vi "SpeedAccelM1.vi"() -> ()   [LabVIEW 2015]
uses:
  <instrlib>/Ion Motion Roboclaw/Ion Motion Roboclaw.lvlib
panel:
  in  "Address":u8
  in  "stop":bool
  in  "Accel":u32(slide) max=800000 step=10000 scale=0.0..800000.0
  in  "Speed":i32(slide)=-40000 min=-40000 max=40000 step=1000 scale=-40000.0..40000.0
  out "Valid":bool
  out "error out":errorcluster
  in  "COM port":refnum<visa-resource-name>
  in  "baud rate (38400)":u32
  in  "error in (no error)":errorcluster
  # "This example assumes the Velocity PID  values have already been tuned for the motor and saved to the Roboclaw."
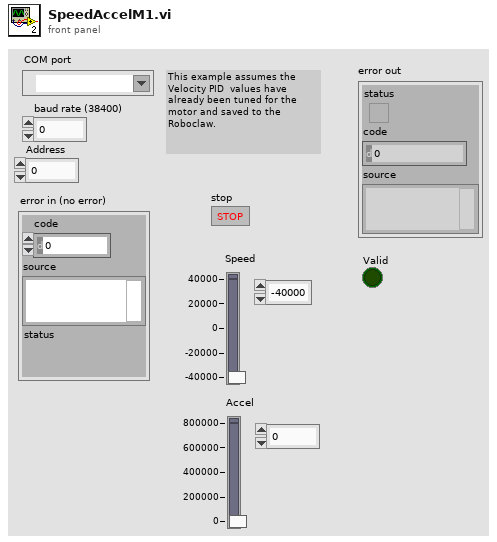
[diagram p1: front panel]
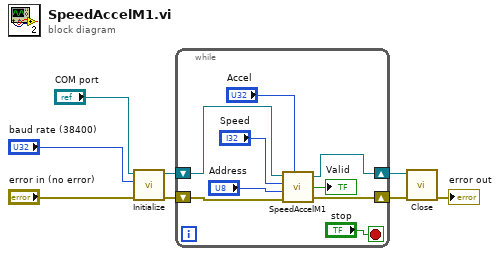
[diagram p0: block diagram]
diagram:
  n1 = call <instrlib>:"Initialize.vi"("error in (no error)"="error in (no error)", "baud rate (38400)"="baud rate (38400)", "COM port"="COM port") -> ("error out"=w7:errorcluster, "VISA resource name out"=w8:refnum<visa-resource-name>)  [unwired: 7 in]
  n2 = while {
    shift-right: [w15] -> w6
    shift-left: w8 -> [w17]
    shift-right: [w14] -> w5
    shift-left: w7 -> [w16]
    stop <- "stop" stop-if-true
    n3 = call <instrlib>:"SpeedAccelM1.vi"("VISA Refnum in"=w17, "Accel"="Accel", "Speed"="Speed", "Address"="Address", "error in (no error)"=w16) -> ("VISA Refnum out"=w15:refnum<visa-resource-name>, "Valid"=→"Valid":bool, "error out"=w14:errorcluster)  [unwired: 1 in]
  }
  n4 = call <instrlib>:"Close.vi"("error in (no error)"=w5, "VISA resource name"=w6) -> ("error out"=→"error out":errorcluster)  [unwired: 9 in]
